vi "Get Block Diagram Windows.vi"() -> (3 "VIs With Open BDs":T1(array[cluster]))   [LabVIEW 2019, in "Window.lvlib"]
doc: "Returns a list of VI references with open block diagrams."
uses:
  _Window/Window.lvlib
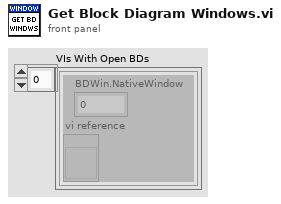
[diagram p1: front panel]
types:
  T1 = cluster{"BDWin.NativeWindow":u64, "vi reference":refnum<vi>}[]
  T2 = typedef "VIMemory VI info.ctl" = cluster{"Project":string, "ComputingNode":string, "VI Name":string, "App Refnum":refnum<vi>}
  T3 = cluster{"BDWin.NativeWindow":u64, "vi reference":refnum<vi>}
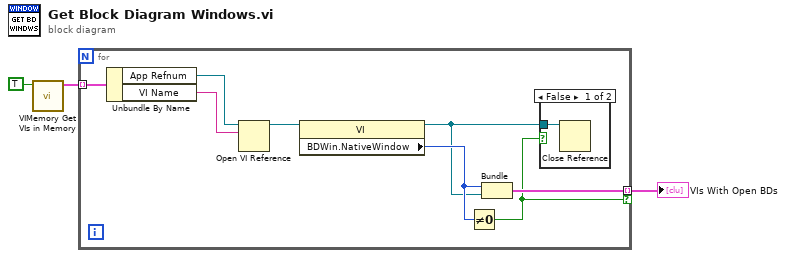
[diagram p0: block diagram]
diagram:
  n1 = call <vilib>:"VIMemory Get VIs in Memory.vi"("Only VIs with Open FPs?"=TRUE) -> ("VIs in memory"=w2:T2[])  [unwired: 9 in, 1 out]
  n2 = for {
    tunnel: [w9] -> w1 mode=indexing if=w4
    tunnel: w2 -> [w8] mode=indexing
    n3 = Unbundle By Name(w8) -> ("App Refnum"=w7:refnum<vi>, "VI Name"=w6:string)
    n4 = Open VI Reference(application reference (local)=w7, vi path=w6) -> (vi reference=w11:refnum<vi>)  [unwired: 4 in, 1 out]
    n5 = property class="VI"(reference=w11) -> (reference out=w5:refnum<vi>, "BDWin.NativeWindow"=w10:u64)  [unwired: 1 in, 1 out]
    n6 = Not Equal To 0?(x=w10) -> (x != 0?=w4:bool)
    n7 = Bundle("BDWin.NativeWindow"=w10, "vi reference"=w5) -> (w9:T3)  [unwired: 1 in]
    n8 = case shown="False" w4 {
      tunnel: w5 -> [w12 _]
      frame False {
        n9 = Close Reference(reference=w12) -> ()  [unwired: 1 in, 1 out]
      }
      frame True {
      }
    }
  }
  "VIs With Open BDs" <- w1
